vi "MakeAndSendInitialOMFJSON.vi"(0 "Allow untrusted certificates?":bool=TRUE, 1 "OMF Producer Token":string, 2 "OMF Ingress URL":string, 5 "OMF Container ID":string, 7 "OMF Static Type ID":string, 9 "OMF Static Type Property Names, Formats, and Values":T3(array[cluster])=[{"Static Property Name"="Data ingress method", "Static Property Format"=enum."string", "Static Property Value"="\"OMF\""}], 11 "OMF Static Type Instance Name":string, 12 "OMF Dynamic Type ID":string, 13 "OMF Dynamic Type Property Names and Formats":T2(array[cluster])=[{"Dynamic Property Name"="X acceleration", "Dynamic Property Format"=enum."string"}, {"Dynamic Property Name"="Y acceleration", "Dynamic Property Format"=enum."string"}, {"Dynamic Property Name"="Z acceleration", "Dynamic Property Format"=enum."string"}]) -> (4 "client handle out":T1, 6 "Reponse headers for initial OMF messages":string, 8 "Response body for initial OMF messages":string, 15 "error out":errorcluster)   [LabVIEW 2021]
uses:
  <vilib>/httpClient/ClientHandle.ctl
  <vilib>/httpClient/LabVIEWHTTPClient.lvlib
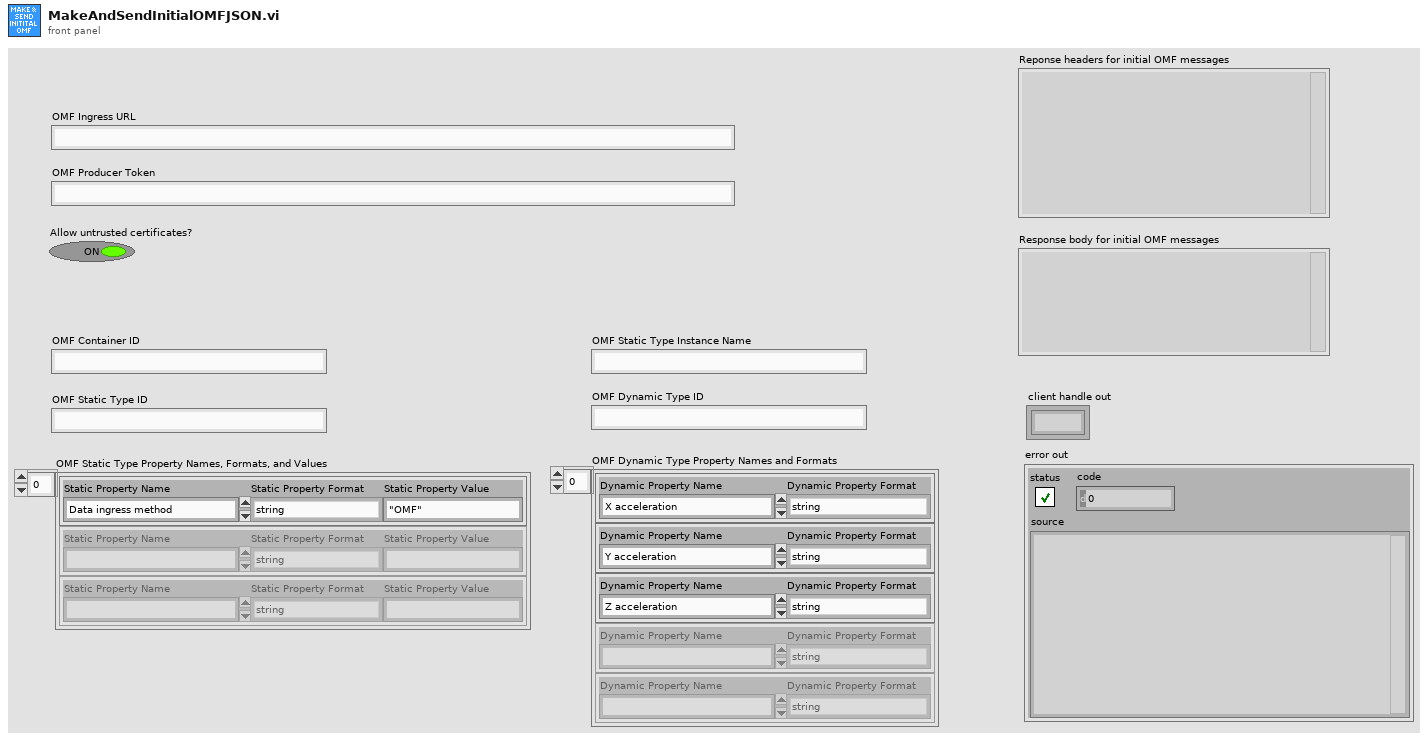
[diagram p1: front panel]
types:
  T1 = typedef "LabVIEWHTTPClient.lvlib/ClientHandle.ctl" = refnum<k1>
  T2 = cluster{"Dynamic Property Name":string, "Dynamic Property Format":enum16{"string", "number"}}[]
  T3 = cluster{"Static Property Name":string, "Static Property Format":enum16{"string", "number"}, "Static Property Value":string}[]
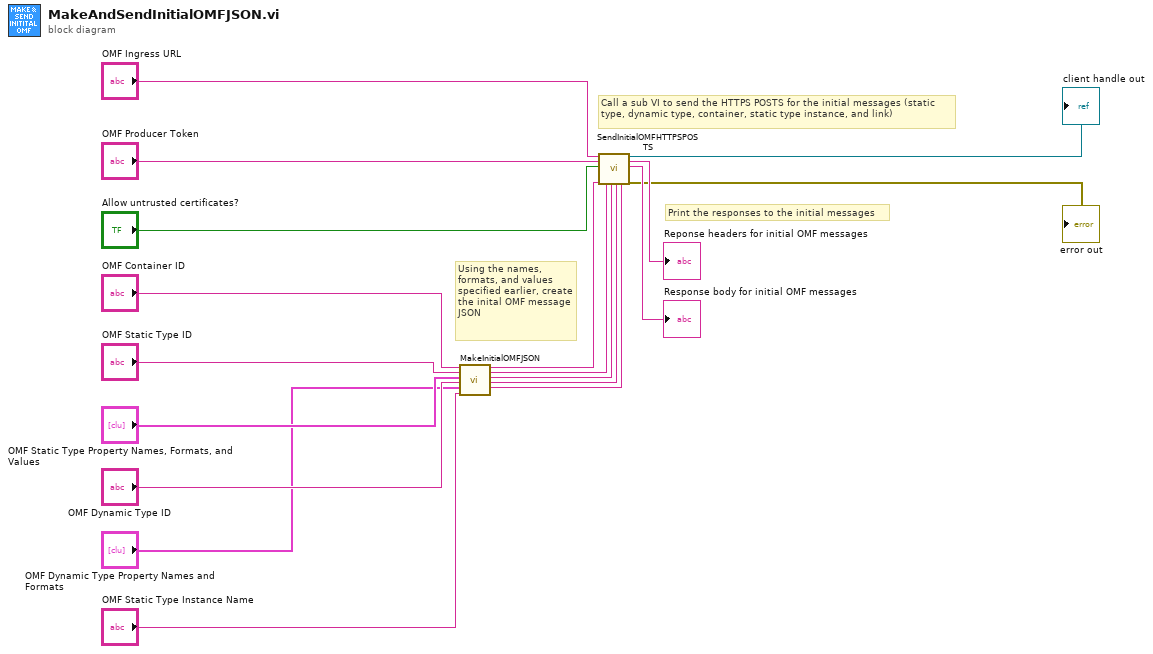
[diagram p0: block diagram]
diagram:
  # "Call a sub VI to send the HTTPS POSTS for the initial messages (static type, dynamic type, container, static type instance, and link)"
  # "Using the names, formats, and values specified earlier, create the inital OMF message JSON"
  # "Print the responses to the initial messages"
  n1 = call "MakeInitialOMFJSON.vi"("OMF Container ID"="OMF Container ID", "OMF Static Type ID"="OMF Static Type ID", "OMF Static Type Property Names, Formats, and Values"="OMF Static Type Property Names, Formats, and Values", "OMF Dynamic Type ID"="OMF Dynamic Type ID", "OMF Dynamic Type Property Names and Formats"="OMF Dynamic Type Property Names and Formats", "OMF Static Type Instance Name"="OMF Static Type Instance Name") -> ("OMF Static Type Message JSON"=w13:string, "OMF Dynamic Type Message JSON"=w12:string, "OMF Container Message JSON"=w11:string, "OMF Static Type Instance Message JSON"=w10:string, "OMF Link Message JSON"=w9:string)  [unwired: 9 in]
  n2 = call "SendInitialOMFHTTPSPOSTS.vi"("OMF Ingress URL"="OMF Ingress URL", "OMF Producer Token"="OMF Producer Token", "Allow untrusted certificates?"="Allow untrusted certificates?", "OMF Static Type Message JSON"=w13, "OMF Dynamic Type Message JSON"=w12, "OMF Container Message JSON"=w11, "OMF Static Type Instance Message JSON"=w10, "OMF Link Message JSON"=w9) -> ("client handle out"=→"client handle out":T1, "Reponse headers for initial OMF messages"=→"Reponse headers for initial OMF messages":string, "Response body for initial OMF messages"=→"Response body for initial OMF messages":string, "error out"=→"error out":errorcluster)  [unwired: 8 in]
